vi "PathPlanner_PathFinder_Key.vi"(8 "Sstart":T1, 9 "G":map{i32, dbl}(c390), 10 "RHS":map{i32, dbl}(c390), 11 "S":T1) -> (3 "DoublePair":T2)   [LabVIEW 2019, in "PathPlanner24.lvlib"]
uses:
  PathPlanner24.lvlib
  PathPlanner_PathFinder_Globals.vi
  TypeDef/PathPlannerFinderDoublePair.ctl
  TypeDef/PathPlannerFinderGridPosition.ctl
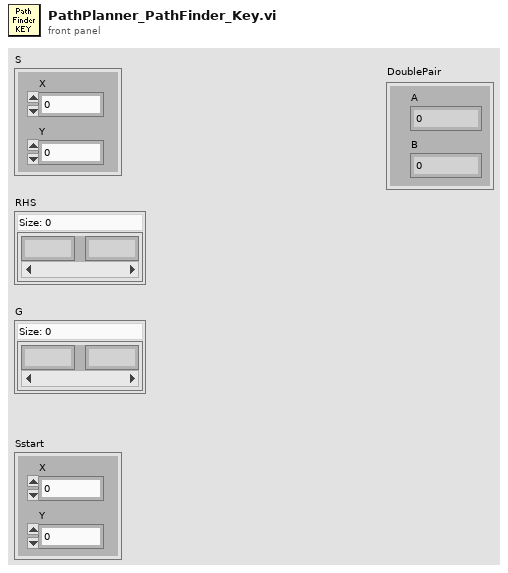
[diagram p1: front panel]
types:
  T1 = typedef "PathPlanner24.lvlib/PathPlannerFinderGridPosition.ctl" = cluster{"X":i32, "Y":i32}
  T2 = typedef "PathPlanner24.lvlib/PathPlannerFinderDoublePair.ctl" = cluster{"A":dbl, "B":dbl}
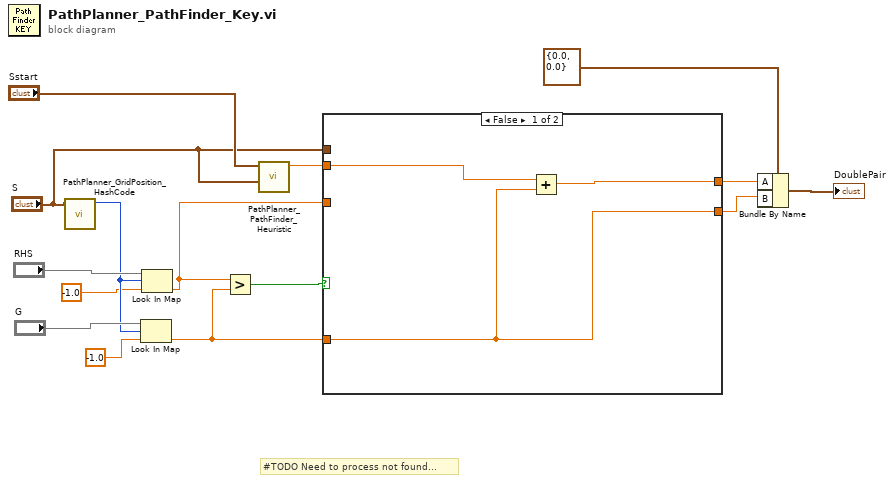
[diagram p0: block diagram]
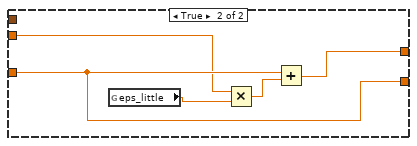
[diagram p2: hidden frame]
diagram:
  # "#TODO Need to process not found..."
  n1 = call "PathPlanner_GridPosition_HashCode.vi"("GridPosition"="S") -> ("HashCode"=w13:i32)  [unwired: 10 in]
  n2 = Look In Map(map="G", key=w13, default value=-1.0) -> (value=w4:dbl)  [unwired: 1 out]
  n3 = Look In Map(map="RHS", key=w13, default value=-1.0) -> (value=w9:dbl)  [unwired: 1 out]
  n4 = Greater?(x=w9, y=w4) -> (0:w10:bool)
  n5 = call "PathPlanner_PathFinder_Heuristic.vi"("sGoal"="S", "sStart"="Sstart") -> ("heuristic"=w3:dbl)  [unwired: 9 in]
  n6 = case shown="False" w10 {
    tunnel: w9 -> [_ w21]
    tunnel: [w18 w23] -> w8
    tunnel: [w17 w21] -> w7
    tunnel: w4 -> [w17 _]
    tunnel: "S" -> [_ _]
    tunnel: w3 -> [w16 w20]
    frame False {
      n7 = Add(x=w16, y=w17) -> (x+y=w18:dbl)
    }
    frame True {
      n8 = global read "PathPlanner_PathFinder_Globals.vi" "eps_little"() -> (w19:dbl)
      n9 = Multiply(x=w20, y=w19) -> (x*y=w22:dbl)
      n10 = Add(x=w21, y=w22) -> (x+y=w23:dbl)
    }
  }
  n11 = Bundle By Name(cluster=T2 {"A"=0.0, "B"=0.0} ("DoublePair"), "A"=w8, "B"=w7) -> (→"DoublePair":T2)
